vi "find channel tag indicies.vi"(10 "channels":refnum<class "TBM channel.lvclass">[](array[class]), 11 "data allocations":T2) -> (3 "classified indices":T1[](array[typedef]))   [LabVIEW 2013, in "control module runtime.lvclass"]
uses:
  control module runtime.lvclass
  <vilib>/NI/Tag Bus Module Framework/channel/data tables.ctl
  <vilib>/NI/Tag Bus/dictionary/data dictionary.lvclass
  <vilib>/NI/Tag Bus/dictionary table pair.ctl
  <vilib>/NI/Tag Bus/table/data table.ctl
  <vilib>/NI/Tag Bus Module Framework/channel/TBM channel.lvclass
  Channel Run Time Mapping Info.ctl
  <vilib>/NI/Tag Bus Module Framework/channel/TBM channel.lvclass/TBM channel.ctl
  <vilib>/NI/Tag Bus/tag/tag descriptor.lvclass/tag descriptor.ctl
  <vilib>/NI/Tag Bus/tag/tag descriptor.lvclass
  <vilib>/NI/Tag Bus/table/data table.lvlib
  <vilib>/NI/Tag Bus/tag bus.lvlib
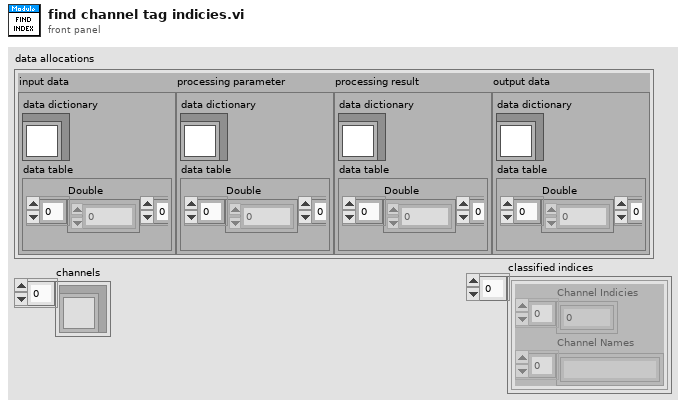
[diagram p1: front panel]
types:
  T1 = typedef "control module runtime.lvclass/Channel Run Time Mapping Info.ctl" = cluster{"Channel Indicies":i32[], "Channel Names":string[]}
  T2 = typedef "TBM channel.lvclass/data tables.ctl" = cluster{"input data":T3, "processing parameter":T3, "processing result":T3, "output data":T3}
  T3 = typedef "tag bus.lvlib/dictionary table pair.ctl" = cluster{"data dictionary":refnum<class "data dictionary.lvclass">, "data table":T4}
  T4 = typedef "tag bus.lvlib/data table.lvlib/data table.ctl" = cluster{"Double":dbl[], "Single":sgl[], "I64":i64[], "I32":i32[], "I16":i16[], "I8":i8[], "U64":u64[], "U32":u32[], "U16":u16[], "U8":u8[], "Boolean":bool[], "String":string[], "Array of Double":cluster{"DBL Array":dbl[]}[], "Array of Single":cluster{"SGL Array":sgl[]}[], "Array of I64":cluster{"I64 Array":i64[]}[], "Array of I32":cluster{"I32 Array":i32[]}[], "Array of I16":cluster{"I16 Array":i16[]}[], "Array of I8":cluster{"I8 Array":i8[]}[], "Array of U64":cluster{"U64 Array":u64[]}[], "Array of U32":cluster{"U32 Array":u32[]}[], "Array of U16":cluster{"U16 Array":u16[]}[], "Array of U8":cluster{"U8 Array":u8[]}[], "Array of Boolean":cluster{"Boolean Array":bool[]}[], "Array of String":cluster{"String Array":string[]}[]}
  T5 = typedef "TBM channel.lvclass/channel classification.ctl" = enum16{"input data", "output data", "processing parameter", "processing result"}
  T6 = typedef "tag bus.lvlib/tag descriptor.lvclass/Data Type.ctl" = enum16{"Double", "Single", "I64", "I32", "I16", "I8", "U64", "U32", "U16", "U8", "Boolean", "String", "Array of Double", "Array of Single", "Array of I64", "Array of I32", "Array of I16", "Array of I8", "Array of U64", "Array of U32", "Array of U16", "Array of U8", "Array of Boolean", "Array of String"}
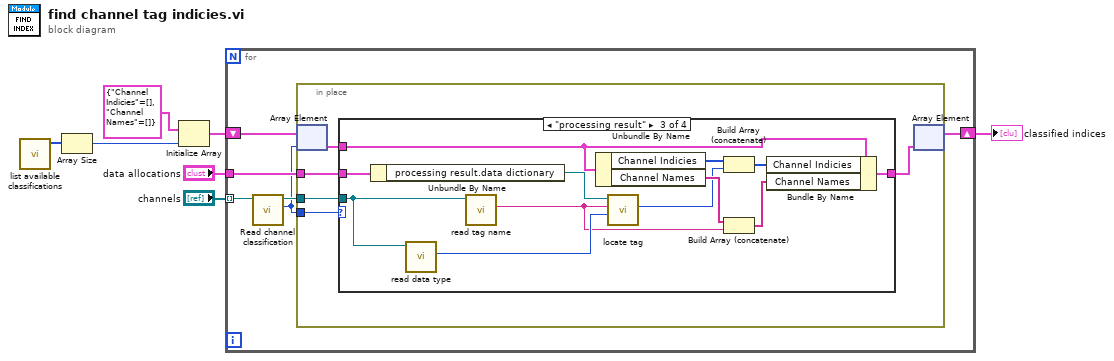
[diagram p0: block diagram]
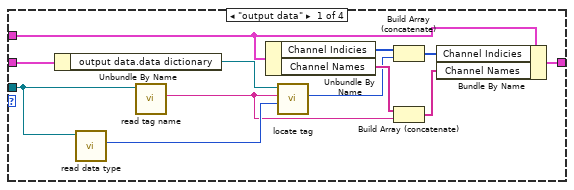
[diagram p2: hidden frame]
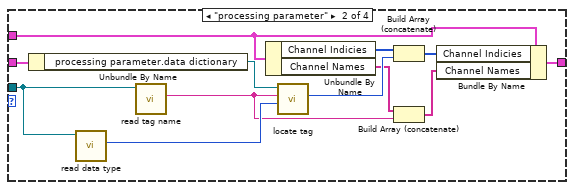
[diagram p3: hidden frame]
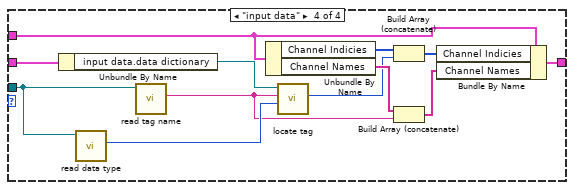
[diagram p4: hidden frame]
diagram:
  n1 = call <vilib>:"list available classifications.vi"() -> ("supported types"=w5:T5[])  [unwired: 11 in]
  n2 = Array Size(array=w5) -> (size(s)=w3:i32)
  n3 = Initialize Array(T1 {"Channel Indicies"=[], "Channel Names"=[]} ("Input Indicies"), w3) -> (w1:T1[])
  n4 = for {
    tunnel: "channels" -> [w13] mode=indexing
    tunnel: "data allocations" -> [w12]
    shift-right: [w8] -> w4
    shift-left: w1 -> [w10]
    n5 = call <vilib>:"Read channel classification.vi"("channel in"=w13) -> ("channel classification"=w9:T5, "channel out"=w11:refnum<class "TBM channel.lvclass">)  [unwired: 8 in, 1 out]
    n6 = in-place {
      in-place-border: w9 -> [w18]
      in-place-border: w12 -> [w17]
      in-place-border: w11 -> [w16]
      n7 = in-place-array #1(w10, w9) -> (w15:T1)
      n8 = case shown="\"processing result\"" w18 {
        tunnel: w17 -> [w30 w42 w54 w66]
        tunnel: w16 -> [w28 w40 w52 w64]
        tunnel: w15 -> [w22 w32 w43 w55]
        tunnel: [w21 w31 w44 w56] -> w14
        frame "output data" {
          n9 = Unbundle By Name(w30) -> ("output data.data dictionary"=w29:refnum<class "data dictionary.lvclass">)
          n10 = call <vilib>:"read data type.vi"("system tag in"=w28) -> ("data type"=w27:T6)  [unwired: 8 in, 2 out]
          n11 = call <vilib>:"read tag name.vi"("system tag in"=w28) -> ("name"=w20:string)  [unwired: 8 in, 2 out]
          n12 = Unbundle By Name(w22) -> ("Channel Indicies"=w24:i32[], "Channel Names"=w26:string[])
          n13 = call <vilib>:"locate tag.vi"("data type"=w27, "name"=w20, "data dictionary in"=w29) -> ("index"=w19:i32)  [unwired: 6 in, 2 out]
          n14 = Build Array (concatenate)(w24, w19) -> (w25:i32[])
          n15 = Build Array (concatenate)(w26, w20) -> (w23:string[])
          n16 = Bundle By Name(cluster=w22, "Channel Indicies"=w25, "Channel Names"=w23) -> (w21:T1)
        }
        frame "processing parameter" {
          n17 = Unbundle By Name(w42) -> ("processing parameter.data dictionary"=w41:refnum<class "data dictionary.lvclass">)
          n18 = call <vilib>:"read data type.vi"("system tag in"=w40) -> ("data type"=w39:T6)  [unwired: 8 in, 2 out]
          n19 = call <vilib>:"read tag name.vi"("system tag in"=w40) -> ("name"=w35:string)  [unwired: 8 in, 2 out]
          n20 = Unbundle By Name(w32) -> ("Channel Indicies"=w37:i32[], "Channel Names"=w36:string[])
          n21 = call <vilib>:"locate tag.vi"("data type"=w39, "name"=w35, "data dictionary in"=w41) -> ("index"=w38:i32)  [unwired: 6 in, 2 out]
          n22 = Build Array (concatenate)(w37, w38) -> (w34:i32[])
          n23 = Build Array (concatenate)(w36, w35) -> (w33:string[])
          n24 = Bundle By Name(cluster=w32, "Channel Indicies"=w34, "Channel Names"=w33) -> (w31:T1)
        }
        frame "processing result" {
          n25 = Unbundle By Name(w54) -> ("processing result.data dictionary"=w53:refnum<class "data dictionary.lvclass">)
          n26 = call <vilib>:"read data type.vi"("system tag in"=w52) -> ("data type"=w51:T6)  [unwired: 8 in, 2 out]
          n27 = call <vilib>:"read tag name.vi"("system tag in"=w52) -> ("name"=w47:string)  [unwired: 8 in, 2 out]
          n28 = Unbundle By Name(w43) -> ("Channel Indicies"=w46:i32[], "Channel Names"=w50:string[])
          n29 = call <vilib>:"locate tag.vi"("data type"=w51, "name"=w47, "data dictionary in"=w53) -> ("index"=w48:i32)  [unwired: 6 in, 2 out]
          n30 = Build Array (concatenate)(w46, w48) -> (w49:i32[])
          n31 = Build Array (concatenate)(w50, w47) -> (w45:string[])
          n32 = Bundle By Name(cluster=w43, "Channel Indicies"=w49, "Channel Names"=w45) -> (w44:T1)
        }
        frame "input data" {
          n33 = Unbundle By Name(w66) -> ("input data.data dictionary"=w65:refnum<class "data dictionary.lvclass">)
          n34 = call <vilib>:"read data type.vi"("system tag in"=w64) -> ("data type"=w63:T6)  [unwired: 8 in, 2 out]
          n35 = call <vilib>:"read tag name.vi"("system tag in"=w64) -> ("name"=w58:string)  [unwired: 8 in, 2 out]
          n36 = Unbundle By Name(w55) -> ("Channel Indicies"=w60:i32[], "Channel Names"=w62:string[])
          n37 = call <vilib>:"locate tag.vi"("data type"=w63, "name"=w58, "data dictionary in"=w65) -> ("index"=w57:i32)  [unwired: 6 in, 2 out]
          n38 = Build Array (concatenate)(w60, w57) -> (w61:i32[])
          n39 = Build Array (concatenate)(w62, w58) -> (w59:string[])
          n40 = Bundle By Name(cluster=w55, "Channel Indicies"=w61, "Channel Names"=w59) -> (w56:T1)
        }
      }
      n41 = in-place-array #1(w14) -> (w8:T1[])  [unwired: 1 out]
    }
  }
  "classified indices" <- w4
